vi "Read Amplitude All.vi"(8 "error in (no error)":errorcluster {"code" format="%.0x"}, 9 "ValBufferSize":i32=2048, 11 "instrument handle":refnum<k15>) -> (0 "error out":errorcluster {"code" format="%.0x"}, 1 "ValActualSize":i32, 2 "Val":dbl[](array[numeric]) format="%.2p", 3 "instrument handle out":refnum<k15>)   [LabVIEW 2009, in "Keysight XSAn.lvlib"]
doc: "Returns the amplitude values of the first 10 harmonics.\n\nSupported Models: M9290A, N8973B, N8974B, N8975B, N8976B, N9000A, N9000B, N9010A, N9010B, N9020A, N9020B, N9030A, N9030B, N9038A, N9040B, N9041B, SPN9003A, SPN9026A"
uses:
  <instrlib>/Keysight XSAn/Keysight XSAn.lvlib
  AgXSAn.dll
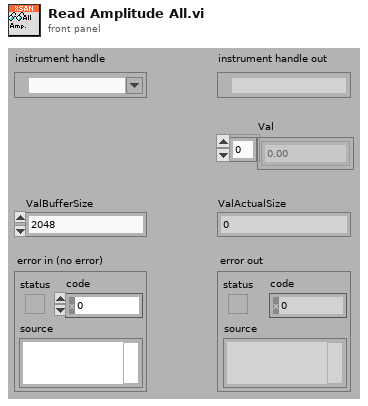
[diagram p1: front panel]
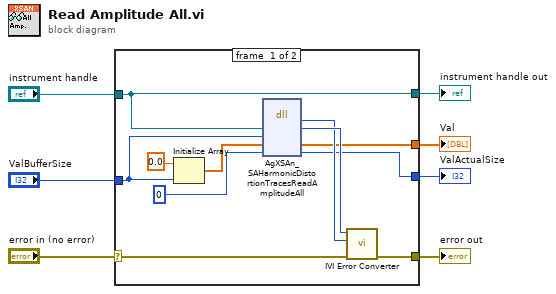
[diagram p0: block diagram]
diagram:
  n1 = case shown="No Error" "error in (no error)" {
    selector: "error in (no error)" -> [w16 w20]
    tunnel: [w15 w20] -> w7
    tunnel: "instrument handle" -> [w9 w19]
    tunnel: "ValBufferSize" -> [w8 _]
    tunnel: [w12 _] -> w3
    tunnel: [w10 _] -> w2
    tunnel: [w9 w19] -> w1
    frame #0 {
      n2 = Initialize Array(0.0 ("element"), w8) -> (w14:dbl[])
      n3 = dll-call lib="AgXSAn**.dll" fn="AgXSAn_SAHarmonicDistortionTracesReadAmplitudeAll"("Vi"=w9, "ValBufferSize"=w8, "Val"=w14, "ValActualSize"=0) -> (w17:i32, "Vi"=w18:u32, "Val"=w12:dbl[], "ValActualSize"=w10:i32)  [unwired: 4 in, 2 out]
      n4 = call <instrlib>:"IVI Error Converter.vi"("error in (no error)"=w16, "IVI error code (0)"=w17, "instrument handle"=w18) -> ("error out"=w15:errorcluster)  [unwired: 7 in, 1 out]
    }
    frame #1 {
    }
  }
  "error out" <- w7
  "instrument handle out" <- w1
  "Val" <- w3
  "ValActualSize" <- w2
